vi "Configure Counter Totalizer Characteristics.vi"(0 "VISA resource name":refnum<visa-resource-name>, 1 "Slope (0: Negative)":i32(ring) items=["Negative", "Positive"], 5 "Enable Totalizer Gating (F: Disable)":bool, 7 "Counter Source (1: Channel 2)":i32(ring)=1 items=["Channel 1", "Channel 2", "Channel 3", "Channel 4"], 9 "Gating Signal Polarity (0: Negative)":i32(ring) items=["Negative", "Positive"], 11 "error in (no error)":errorcluster) -> (4 "VISA resource name out":refnum<visa-resource-name>, 15 "error out":errorcluster)   [LabVIEW 2015, in "Agilent 2000 3000 X-Series.lvlib"]
doc: "Configures the totalize mode for the counter. \n\n<b>Note:</b>\nOnly supported by the 3000 T Series models."
uses:
  Agilent 2000 3000 X-Series.lvlib
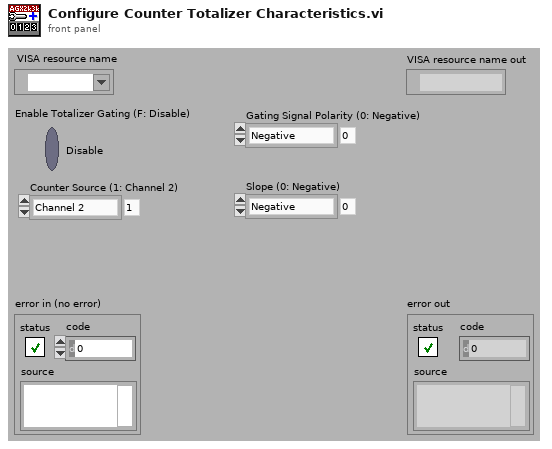
[diagram p1: front panel]
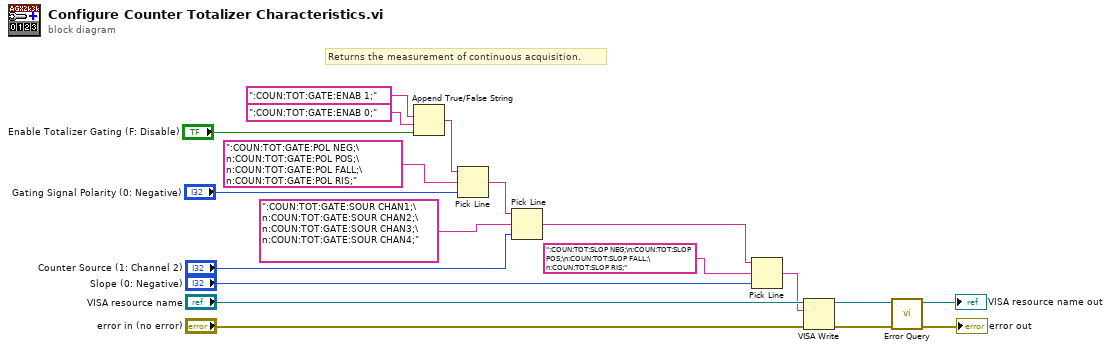
[diagram p0: block diagram]
diagram:
  # "Returns the measurement of continuous acquisition."
  n1 = Append True/False String(1:"Enable Totalizer Gating (F: Disable)", 2:":COUN:TOT:GATE:ENAB 0;" ("false string"), 3:":COUN:TOT:GATE:ENAB 1;" ("true string")) -> (0:w8:string)  [unwired: 1 in]
  n2 = Pick Line(string ("")=w8, multi-line string=":COUN:TOT:GATE:POL NEG;\n:COUN:TOT:GATE:POL POS;\n:COUN:TOT:GATE:POL FALL;\n:COUN:TOT:GATE:POL RIS;", line index="Gating Signal Polarity (0: Negative)") -> (output string=w7:string)
  n3 = Pick Line(string ("")=w7, multi-line string=":COUN:TOT:GATE:SOUR CHAN1;\n:COUN:TOT:GATE:SOUR CHAN2;\n:COUN:TOT:GATE:SOUR CHAN3;\n:COUN:TOT:GATE:SOUR CHAN4;", line index="Counter Source (1: Channel 2)") -> (output string=w3:string)
  n4 = Pick Line(string ("")=w3, multi-line string=":COUN:TOT:SLOP NEG;\n:COUN:TOT:SLOP POS;\n:COUN:TOT:SLOP FALL;\n:COUN:TOT:SLOP RIS;", line index="Slope (0: Negative)") -> (output string=w1:string)
  n5 = VISA Write(VISA resource name="VISA resource name", write buffer=w1, error in (no error)="error in (no error)") -> (VISA resource name out=w17:refnum<visa-resource-name>, error out=w16:errorcluster)  [unwired: 1 out]
  n6 = call "Error Query.vi"("error in (no error)"=w16, "VISA resource name"=w17) -> ("error out"=→"error out":errorcluster, "VISA resource name out"=→"VISA resource name out":refnum<visa-resource-name>)  [unwired: 8 out]
